vi "SLM_Grating.vi"(2 "y angle (mrad)":dbl, 3 "x angle (mrad)":dbl, 4 "wavelength":dbl) -> (0 "k y":dbl, 1 "k x":dbl)   [LabVIEW 2024]
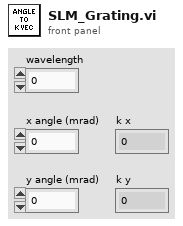
[diagram p1: front panel]
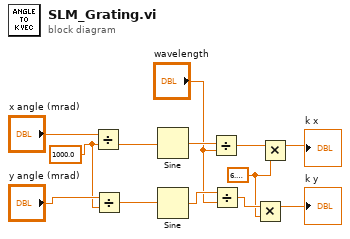
[diagram p0: block diagram]
diagram:
  w1 = 6.283185307179586
  w8 = 1000.0 ("y")
  n1 = Divide(x="x angle (mrad)", y=w8) -> (x/y=w11:dbl)
  n2 = Divide(x="y angle (mrad)", y=w8) -> (x/y=w7:dbl)
  n3 = Sine(x=w11) -> (sin(x)=w6:dbl)
  n4 = Sine(x=w7) -> (sin(x)=w5:dbl)
  n5 = Divide(x=w6, y="wavelength") -> (x/y=w13:dbl)
  n6 = Divide(x=w5, y="wavelength") -> (x/y=w12:dbl)
  n7 = Multiply(x=w12, y=w1) -> (x*y=→"k y":dbl)
  n8 = Multiply(x=w13, y=w1) -> (x*y=→"k x":dbl)
